vi "SET_RTC_TIME.vi"(8 "error in (no error)":errorcluster, 11 "New Time":timestamp=timestamp(2082805200 s since 1904-01-01)) -> (0 "error out":errorcluster)   [LabVIEW 2019]
uses:
  Typedefs/Message.ctl
  Typedefs/Sensor Types.ctl
  Typedefs/Message Types.ctl
  Message Globals.vi
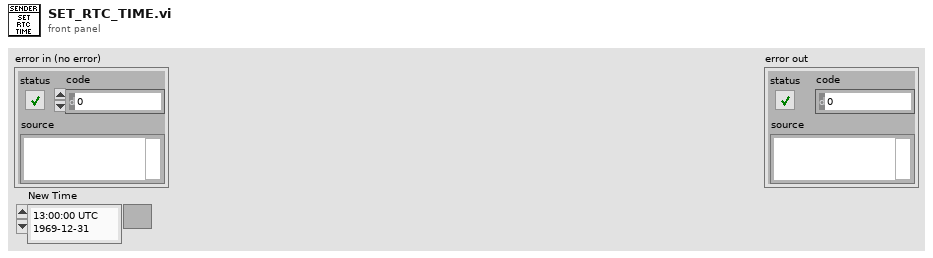
[diagram p1: front panel]
types:
  T1 = typedef "Message Types.ctl" = enum16{"HEART_BEAT", "CONNECT", "GET_CURRENT_MEASUREMENTS", "GET_LOG_FILE", "SEND_LOG_FILE_SIZE", "SEND_LOG_FILE_CHUNK", "GET_LOGGING_PERIOD", "SET_LOGGING_PERIOD", "SEND_SD_CARD_INFO", "GET_LOGS_LIST", "SEND_LOG_FILE_NAME", "SEND_LOGGING_PERIOD", "GET_RTC_TIME", "SET_RTC_TIME", "SEND_RTC_TIME", "SEND_CURRENT_MEASUREMENTS", "DELETE_LOG_FILE", "GET_SD_CARD_INFO", "GET_BATTERY_INFO", "SEND_BATTERY_INFO", "GET_LOG_FILE_SIZE", "SET_WIFI_SSID", "SET_WIFI_PASSWORD", "GET_WIFI_DETAILS", "SEND_WIFI_DETAILS", "ERROR_MSG"}
  T2 = typedef "Message.ctl" = cluster{"Payload Size":u8, "Sequence Number":u8, "Sensor Type":T3, "Message Types":T1, "Data":u8[]}
  T3 = typedef "Sensor Types.ctl" = enum16{"APP", "TURBIDITY", "PH"}
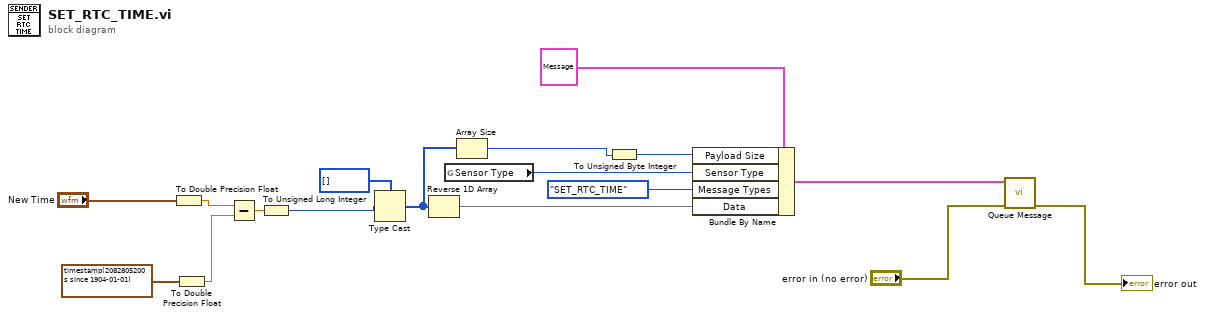
[diagram p0: block diagram]
diagram:
  n1 = To Double Precision Float(number="New Time") -> (double precision float=w9:dbl)
  n2 = To Double Precision Float(number=timestamp(2082805200 s since 1904-01-01)) -> (double precision float=w10:dbl)
  n3 = Subtract(x=w9, y=w10) -> (x-y=w8:dbl)
  n4 = To Unsigned Long Integer(number=w8) -> (unsigned 32bit integer=w5:u32)
  n5 = Type Cast(type=u8[] [], x=w5) -> (*(type *) &x=w3:u8[])
  n6 = Reverse 1D Array(array=w3) -> (reversed array=w4:u8[])
  n7 = global read "Message Globals.vi" "Sensor Type"() -> (w15:T3)
  n8 = Array Size(array=w3) -> (size(s)=w1:i32)
  n9 = To Unsigned Byte Integer(number=w1) -> (unsigned 8bit integer=w2:u8)
  n10 = Bundle By Name(cluster=T2 {"Payload Size"=0, "Sequence Number"=0, "Sensor Type"=enum."APP", "Message Types"=enum."HEART_BEAT", "Data"=[]} ("Message"), "Payload Size"=w2, "Sensor Type"=w15, "Message Types"=Message_Types."SET_RTC_TIME", "Data"=w4) -> (w14:T2)
  n11 = call "Queue Message.vi"("error in (no error)"="error in (no error)", "Message"=w14) -> ("error out"=→"error out":errorcluster)  [unwired: 9 in]
